vi "begin stream read until termination.vi"(5 "id":u32, 7 "event":refnum<user-event>, 8 "error in":errorcluster, 9 "max bytes":u32, 10 "termination":string, 11 "socket":u64) -> (0 "error out":errorcluster)   [LabVIEW 2016, in "async tls dl.lvlib"]
uses:
  async tls dl.lvlib
  action complete event.ctl
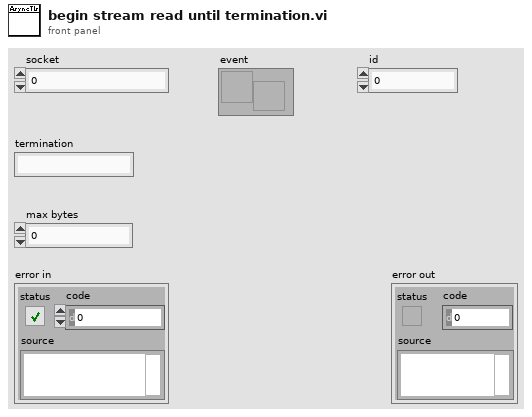
[diagram p1: front panel]
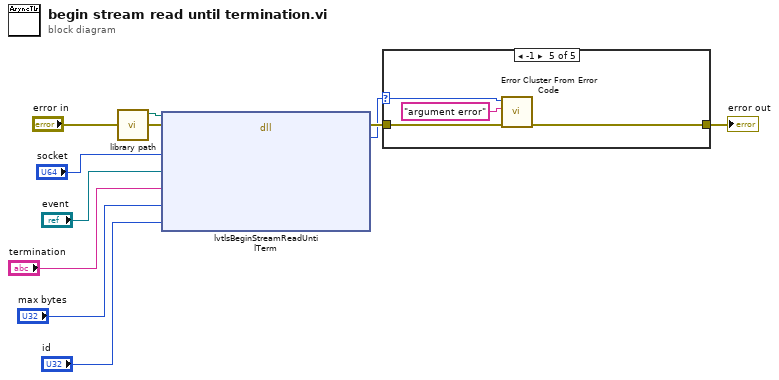
[diagram p0: block diagram]
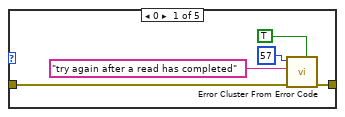
[diagram p2: hidden frame]
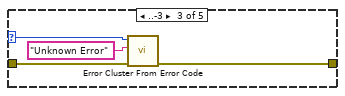
[diagram p4: hidden frame]
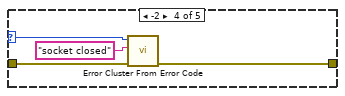
[diagram p5: hidden frame]
diagram:
  n1 = call "library path.vi"() -> ("path"=w4:path)  [unwired: 11 in]
  n2 = dll-call lib="C:/Users/IEUser/Desktop/libasynclvtls/lvasynctls.dll" fn="lvtlsBeginStreamReadUntilTerm"(path in=w4, error in="error in", "socket"="socket", "event"="event", "termination"="termination", "bytes to read"="max bytes", "id"="id") -> (error out=w2:errorcluster, "err"=w1:i32)  [unwired: 6 in, 1 out]
  n3 = case shown="-1" w1 {
    selector: w1 -> [_ _ w19 w23 w27]
    tunnel: w2 -> [w14 w16 w20 w24 w28]
    tunnel: [w15 w16 w18 w22 w26] -> w3
    frame 0 {
      n4 = call <vilib>:"Error Cluster From Error Code.vi"("is warning? (False)"=TRUE, "error in (no error)"=w14, "error message (\"\")"="try again after a read has completed" ("error message (\"\")"), "error code (0)"=57) -> ("error out"=w15:errorcluster)  [unwired: 5 in]
    }
    frame 1.. {
    }
    frame ..-3 {
      n5 = call <vilib>:"Error Cluster From Error Code.vi"("error in (no error)"=w20, "error message (\"\")"="Unknown Error" ("error message (\"\")"), "error code (0)"=w19) -> ("error out"=w18:errorcluster)  [unwired: 6 in]
    }
    frame -2 {
      n6 = call <vilib>:"Error Cluster From Error Code.vi"("error in (no error)"=w24, "error message (\"\")"="socket closed" ("error message (\"\")"), "error code (0)"=w23) -> ("error out"=w22:errorcluster)  [unwired: 6 in]
    }
    frame -1 {
      n7 = call <vilib>:"Error Cluster From Error Code.vi"("error in (no error)"=w28, "error message (\"\")"="argument error" ("error message (\"\")"), "error code (0)"=w27) -> ("error out"=w26:errorcluster)  [unwired: 6 in]
    }
  }
  "error out" <- w3
